vi "DBC Sync CAN Msg To Value.vi"(9 "MsgLen":i32, 10 "pCANMsg":u32, 11 "DBCHandle":cluster{}) -> (2 "pCANMsg out":u32, 3 "function return":i32)   [LabVIEW 2010, in "dbc_parser.lvlib"]
doc: "int WINAPI DBC_SyncCANMsgToValue(long long DBCHandle, void* pCANMsg,int MsgLen);"
uses:
  dbc_parser.lvlib
  USB2XXX/trunk/USB2XXX/USB2XXX/vs2019/Release/USB2XXX.dll
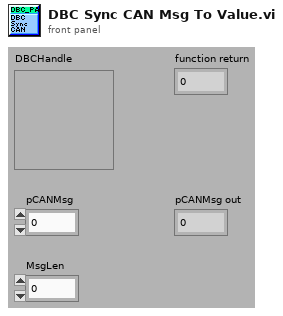
[diagram p1: front panel]
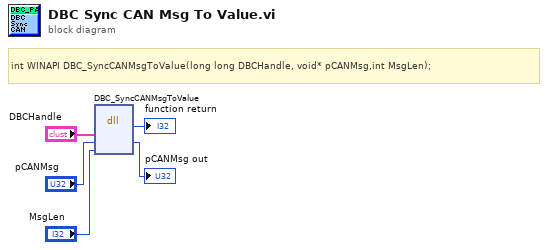
[diagram p0: block diagram]
diagram:
  # "int WINAPI DBC_SyncCANMsgToValue(long long DBCHandle, void* pCANMsg,int MsgLen);"
  n1 = dll-call lib="E:/Projects/USB2XXX/trunk/USB2XXX/USB2XXX/vs2019/Release/USB2XXX.*" fn="DBC_SyncCANMsgToValue"("DBCHandle"="DBCHandle", "pCANMsg"="pCANMsg", "MsgLen"="MsgLen") -> (→"function return":i32, "pCANMsg"=→"pCANMsg out":u32)  [unwired: 5 in, 2 out]
